vi "Append Relative Path String.vi"(8 "Error In":errorcluster, 10 "Relative Path":string, 11 "Base Path":path) -> (0 "Error Out":errorcluster, 3 "Absolute Path":path)   [LabVIEW 2020, in "LMH-Toolbox.lvlib"]
doc: "Build an absolute path from a bath path and a relative path string. \nThis VI strips slashes from relative path and there is platform agnostic."
uses:
  LMH-Toolbox.lvlib
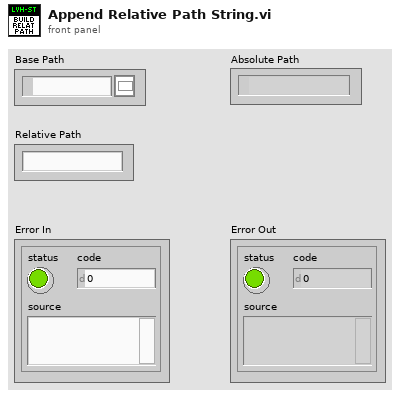
[diagram p1: front panel]
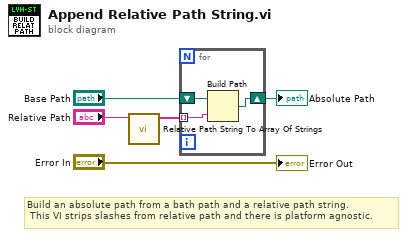
[diagram p0: block diagram]
diagram:
  # "Build an absolute path from a bath path and a relative path string. \n This VI strips slashes from relative path and there is platform agnostic."
  n1 = call "Relative Path String To Array Of Strings.vi"("Relative Path"="Relative Path") -> ("Relative Path Array"=w3:string[])  [unwired: 10 in]
  n2 = for {
    shift-right: [w6] -> w2
    shift-left: "Base Path" -> [w8]
    tunnel: w3 -> [w7] mode=indexing
    n3 = Build Path(base path=w8, name or relative path=w7) -> (appended path=w6:path)
  }
  "Absolute Path" <- w2
  "Error Out" <- "Error In"
